vi "Initialize Waveforms V4.vi"(0 "Image Acquisition Parameters":T2={"Scan Type"=enum."Sample Scanning", "Scan Mode"=enum."XY", "Fast Axis Frequency (Hz)"=100.0, "Image Format"=128, "Line Accumulations"=1, "Frames Per Capture"=1, "Frames Accumulations"=1, "Image Dimension (um)"=[], "Number of Z Steps"=1, "Z Steps Size (um)"=1.0, "Pixel Size (nm)"=[]} {"Z Steps Size (um)" min=0.0; "Number of Z Steps" min=1; "Frames Accumulations" min=1; "Frames Per Capture" min=1; "Line Accumulations" min=1; "Image Format" items=["64 x 64"=64, "128 x 128"=128, "256 x 256"=256, "512 x 512"=512, "1024 x 1024"=1024, "2048 x 2048"=2048]}) -> (4 "Waveform Data to FPGA":T1)   [LabVIEW 2016]
uses:
  Type Defs/Image Acquisition Parameters.ctl
  Waveform Data.ctl
panel:
  in  "Slow Axis 2 Delay (Galvo - Not YZ)":i32=2
  in  "Number Data of Points":i32=5000
  # "Copyright (C) 2020 Edward S Allgeyer\n\nRedistribution and use in source and binary forms, with or without\nmodification, are permitted provided that the following conditions\nare met:\n\n1. Redistributions of source code must retain the above copyright\n   notice, this list of conditions and the following disclaimer.\n\n2. Redistributions in binary form must reproduce the above copyright\n   notice, this list of conditions and the following disclaimer in\n   the documentation and/or other materials provided with the\n   distribution.\n\n3. Neither the name of the copyright holder nor the names of its\n   contributors may be used to endorse or promote products derived\n   from this software without specific prior written permission.\n\nTHIS SOFTWARE IS PROVIDED BY THE COPYRIGHT HOLDERS AND CONTRIBUTORS\n\"AS IS\" AND ANY EXPRESS OR IMPLIED WARRANTIES, INCLUDING, BUT NOT\nLIMITED TO, THE IMPLIED WARRANTIES OF MERCHANTABILITY AND FITNESS\nFOR A PARTICULAR PURPOSE ARE DISCLAIMED. IN NO EVENT SHALL THE\nCOPYRIGHT HOLDER OR CONTRIBUTORS BE LIABLE FOR ANY DIRECT, INDIRECT,\nINCIDENTAL, SPECIAL, EXEMPLARY, OR CONSEQUENTIAL DAMAGES (INCLUDING,\nBUT NOT LIMITED TO, PROCUREMENT OF SUBSTITUTE GOODS OR SERVICES;\nLOSS OF USE, DATA, OR PROFITS; OR BUSINESS INTERRUPTION) HOWEVER\nCAUSED AND ON ANY THEORY OF LIABILITY, WHETHER IN CONTRACT, STRICT\nLIABILITY, OR TORT (INCLUDING NEGLIGENCE OR OTHERWISE) ARISING IN\nANY WAY OUT OF THE USE OF THIS SOFTWARE, EVEN IF ADVISED OF THE\nPOSSIBILITY OF SUCH DAMAGE."
  # "XY"
  # "Z"
  # "Length"
  # "Height"
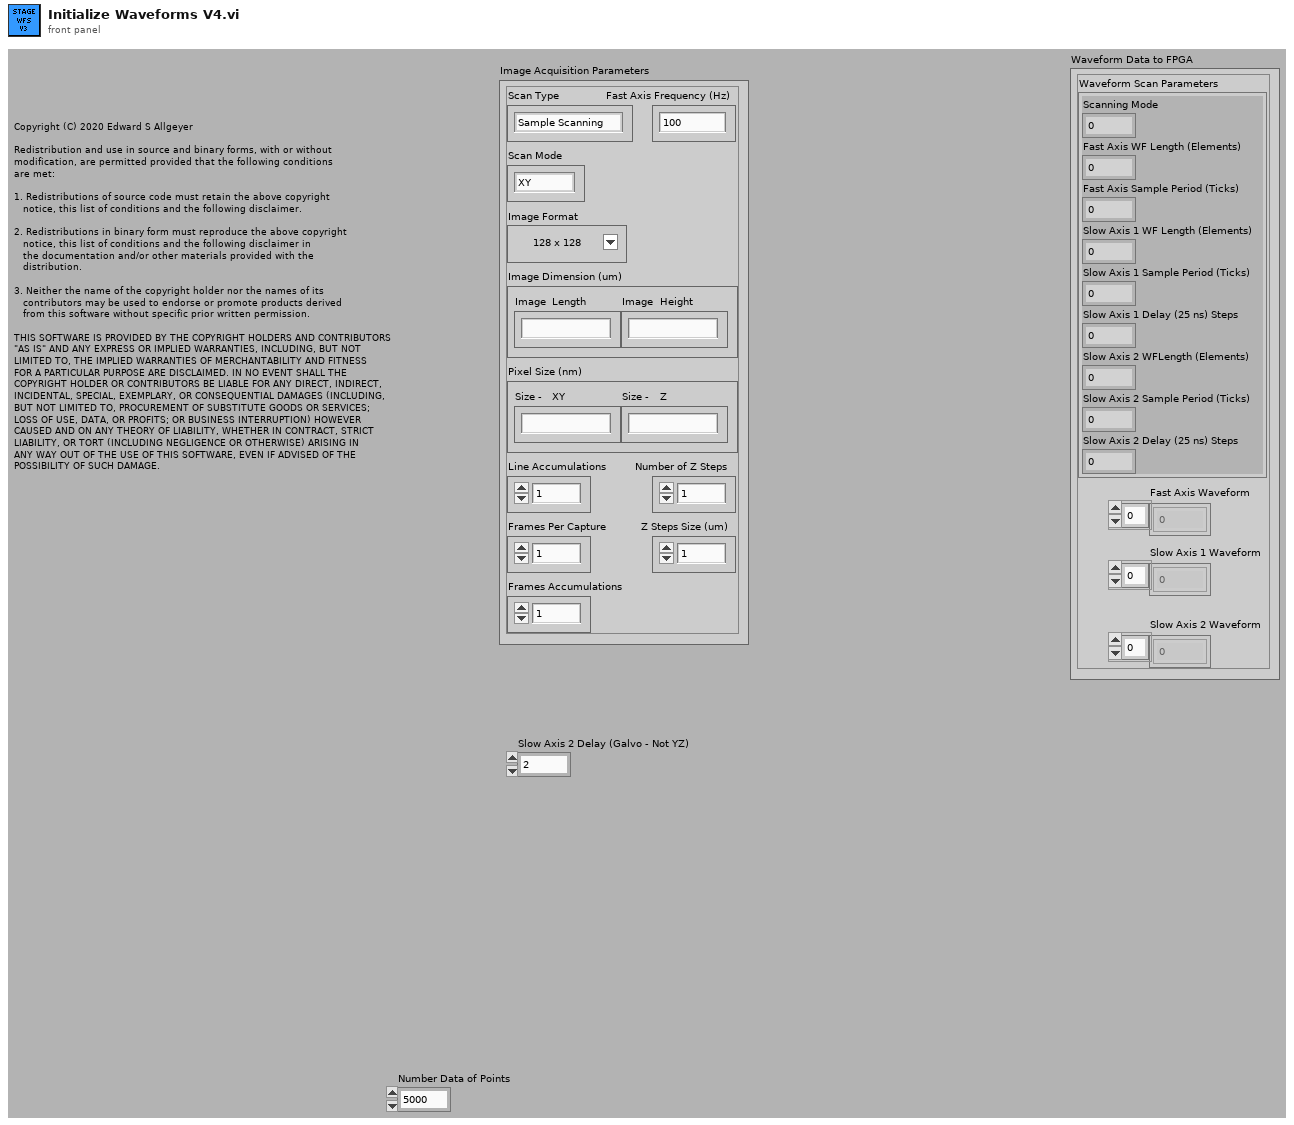
[diagram p1: front panel]
types:
  T1 = typedef "Waveform Data.ctl" = cluster{"Waveform Scan Parameters":cluster{"Scanning Mode":u8, "Fast Axis WF Length (Elements)":i32, "Fast Axis Sample Period (Ticks)":u32, "Slow Axis 1 WF Length (Elements)":i32, "Slow Axis 1 Sample Period (Ticks)":u32, "Slow Axis 1 Delay (25 ns) Steps":i32, "Slow Axis 2 WFLength (Elements)":i32, "Slow Axis 2 Sample Period (Ticks)":u32, "Slow Axis 2 Delay (25 ns) Steps":i32}, "Fast Axis Waveform":dbl[], "Slow Axis 1 Waveform":dbl[], "Slow Axis 2 Waveform":dbl[]}
  T2 = typedef "Image Acquisition Parameters.ctl" = cluster{"Scan Type":enum16{"Sample Scanning", "Beam Scanning"}, "Scan Mode":enum16{"XY", "XZ", "YZ", "XYZ"}, "Fast Axis Frequency (Hz)":dbl, "Image Format":u16, "Line Accumulations":u16, "Frames Per Capture":u16, "Frames Accumulations":u16, "Image Dimension (um)":dbl[], "Number of Z Steps":u8, "Z Steps Size (um)":dbl, "Pixel Size (nm)":dbl[]}
  T3 = cluster{"Scanning Mode":u8, "Fast Axis WF Length (Elements)":i32, "Fast Axis Sample Period (Ticks)":u32, "Slow Axis 1 WF Length (Elements)":i32, "Slow Axis 1 Sample Period (Ticks)":u32, "Slow Axis 1 Delay (25 ns) Steps":i32, "Slow Axis 2 WFLength (Elements)":i32, "Slow Axis 2 Sample Period (Ticks)":u32, "Slow Axis 2 Delay (25 ns) Steps":i32}
  T4 = typedef "Scan Parameters.ctl" = cluster{"Fast_Ax_Amp_V":dbl, "Fast_Ax_Off_V":dbl, "Slow_Ax_Amp_V":dbl, "Slow_Ax_Off_V ":dbl, "Slow_Ax_Max_V_VperS":dbl, "Slow_Ax1_Del25ns":i32, "Slow_Ax2_Del25ns":i32, "Stage_X_Off_V":dbl, "Stage_Y_Off_V":dbl, "Stage_Z_Off_V":dbl, "Galvo1_Off_V":dbl, "Galvo2_Off_V":dbl, "Last_Scan_Mode":enum16{"XY", "XZ", "YZ", "XYZ"}, "Current_Scan_Mode":enum16{"XY", "XZ", "YZ", "XYZ"}, "Fly_Back_Lines":u16, "Linear_Ramp_End":u32, "Z_Step_I16":i16, "Z_Start_I16":i16, "Laser_States _U32":u32, "590_Voltage_I16":i16, "775_AOM_Volt_I16":i16, "Blanking OFF":bool, "Unused_Axis_I16":i16}
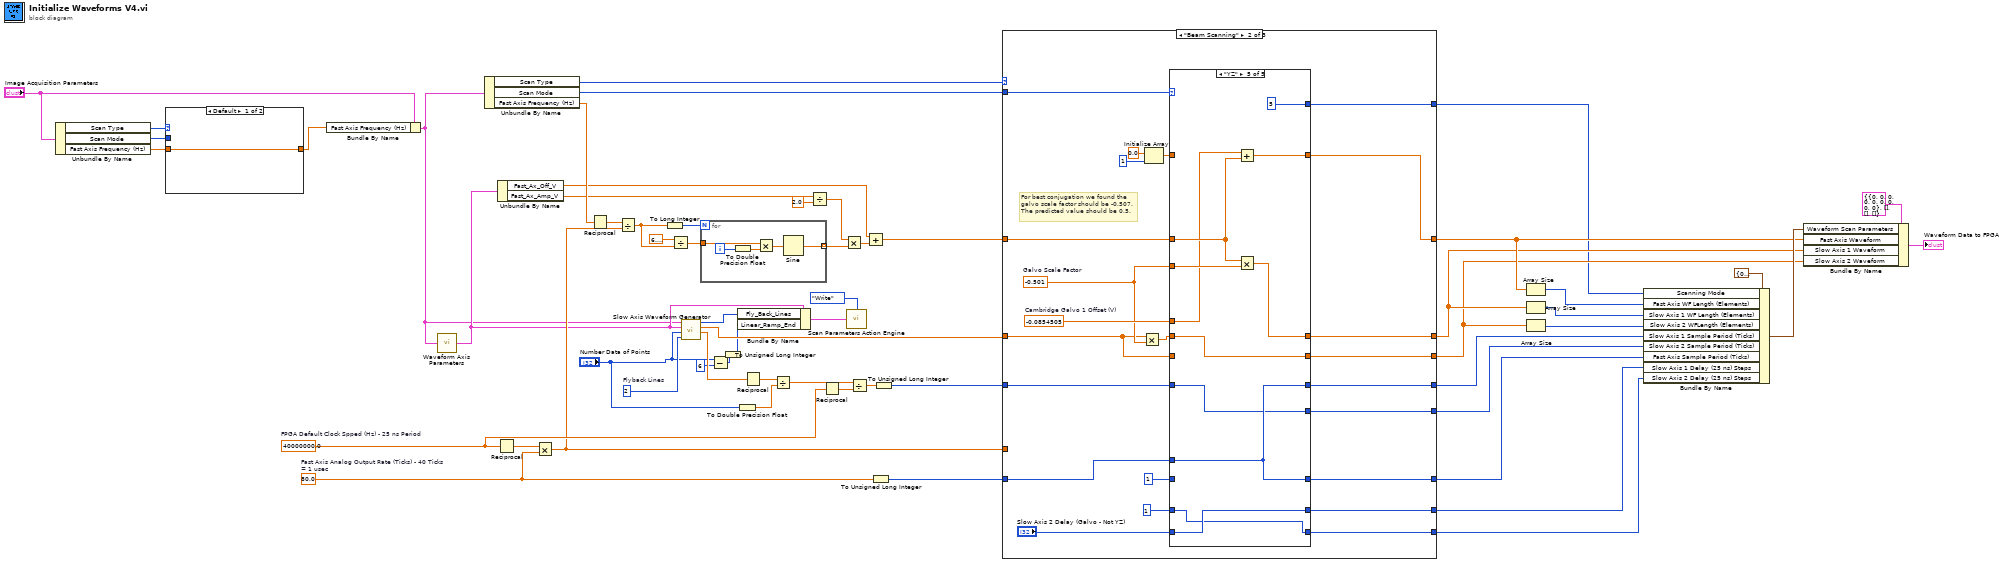
[diagram p0: block diagram]
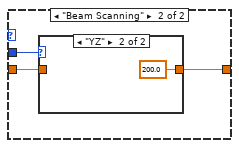
[diagram p2: hidden frame]
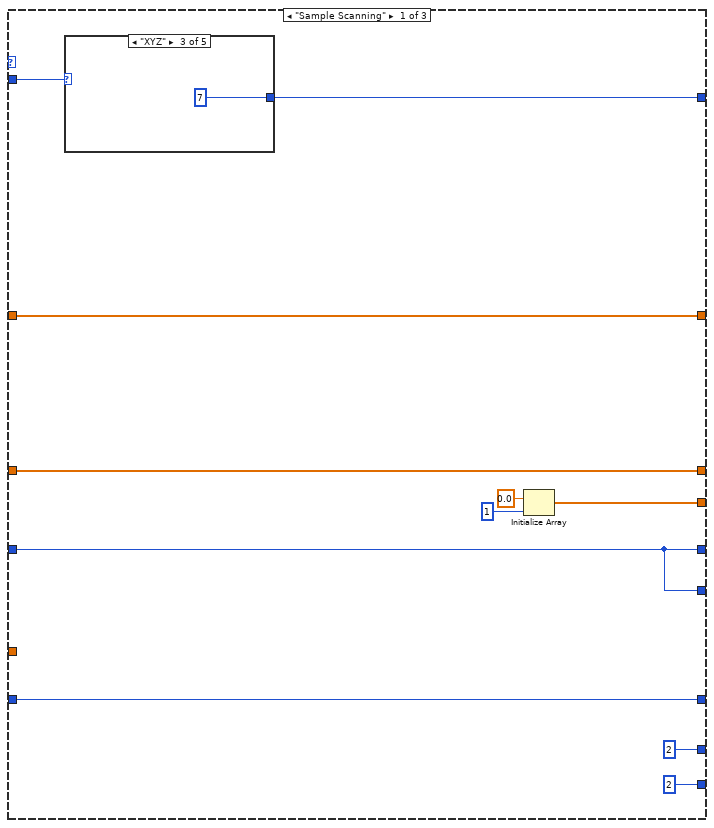
[diagram p4: hidden frame]
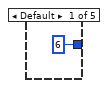
[diagram p5: hidden frame]
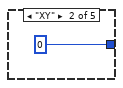
[diagram p6: hidden frame]
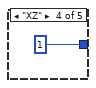
[diagram p7: hidden frame]
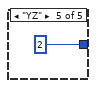
[diagram p8: hidden frame]
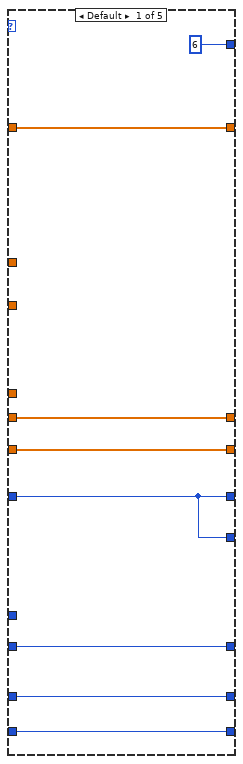
[diagram p9: hidden frame]
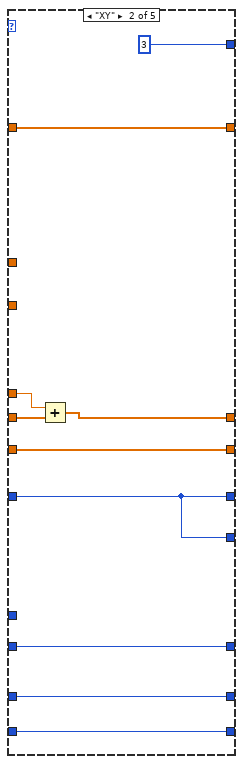
[diagram p10: hidden frame]
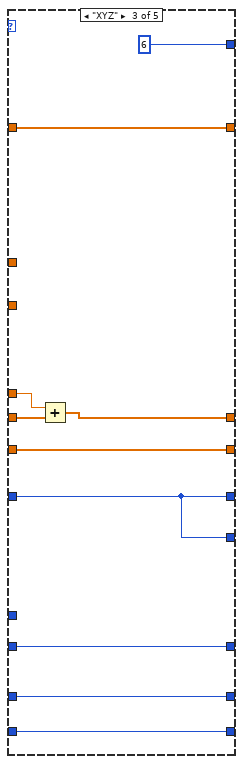
[diagram p11: hidden frame]
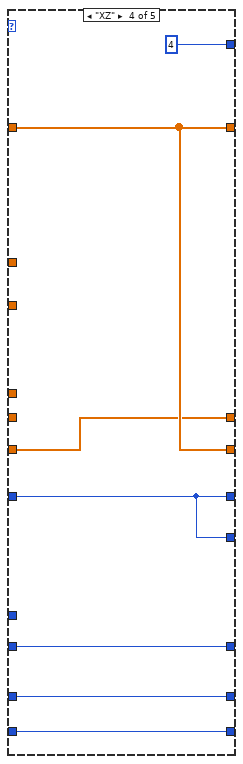
[diagram p12: hidden frame]
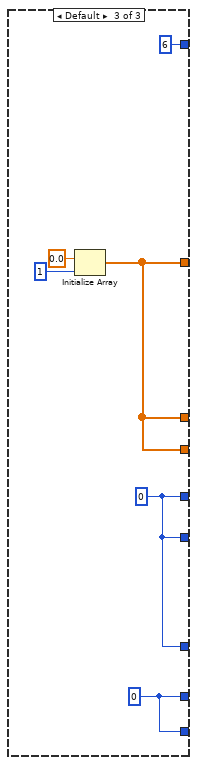
[diagram p13: hidden frame]
diagram:
  w51 = u16 2  # Flyback Lines
  w35 = 80.0  # Fast Axis Analog Output Rate (Ticks) - 40 Ticks = 1 usec
  w45 = 40000000.0  # FPGA Default Clock Spped (Hz) - 25 ns Period
  n1 = Unbundle By Name("Image Acquisition Parameters") -> ("Scan Type"=w10:enum16{"Sample Scanning", "Beam Scanning"}, "Scan Mode"=w9:enum16{"XY", "XZ", "YZ", "XYZ"}, "Fast Axis Frequency (Hz)"=w8:dbl)
  n2 = case shown="Default" w10 {
    tunnel: w9 -> [_ w63]
    tunnel: [w60 w61] -> w7
    tunnel: w8 -> [w60 w62]
    frame Default {
    }
    frame "Beam Scanning" {
      n3 = case shown="\"YZ\"" w63 {
        tunnel: [w64 200.0 ("Fast Axis Frequency (Hz)")] -> w61
        tunnel: w62 -> [w64 _]
        frame Default {
        }
        frame "YZ" {
        }
      }
    }
  }
  n4 = Bundle By Name(cluster="Image Acquisition Parameters", "Fast Axis Frequency (Hz)"=w7) -> (w5:T2)
  n5 = call "Waveform Axis Parameters.vi"("Image Acquisition Parameters"=w5) -> ("Scan Parameters"=w11:T4)  [unwired: 14 in]
  n6 = Unbundle By Name(w5) -> ("Scan Type"=w50:enum16{"Sample Scanning", "Beam Scanning"}, "Scan Mode"=w49:enum16{"XY", "XZ", "YZ", "XYZ"}, "Fast Axis Frequency (Hz)"=w20:dbl)
  n7 = Unbundle By Name(w11) -> ("Fast_Ax_Off_V"=w17:dbl, "Fast_Ax_Amp_V"=w18:dbl)
  n8 = Reciprocal(x=w45) -> (1/x=w48:dbl)
  n9 = Multiply(x=w48, y=w35) -> (x*y=w15:dbl)
  n10 = Reciprocal(x=w20) -> (1/x=w25:dbl)
  n11 = Divide(x=w25, y=w15) -> (x/y=w23:dbl)
  n12 = To Long Integer(number=w23) -> (32bit integer=w24:i32)
  n13 = Divide(x=6.283185307179586, y=w23) -> (x/y=w28:dbl)
  n14 = call "Slow Axis Waveform Generator.vi"("Flyback Lines"=w51, "Number Data of Points"="Number Data of Points", "Scan Parameters"=w11, "Image Acquisition Parameters"=w5) -> ("Slow Axis Frequency"=w46:dbl, "Slow Axis Waveform"=w47:dbl[], "Flyback Lines"=w14:u16)  [unwired: 1 out]
  n15 = for {
    N: w24 -> [_]
    tunnel: w28 -> [w70]
    tunnel: [w67] -> w27 mode=indexing
    i -> [w66]
    n16 = To Double Precision Float(number=w66) -> (double precision float=w69:dbl)
    n17 = Multiply(x=w70, y=w69) -> (x*y=w68:dbl)
    n18 = Sine(x=w68) -> (sin(x)=w67:dbl)
  }
  n19 = Subtract(x="Number Data of Points", y=6) -> (x-y=w2:i32)
  n20 = To Unsigned Long Integer(number=w2) -> (unsigned 32bit integer=w1:u32)
  n21 = Bundle By Name(cluster=w11, "Fly_Back_Lines"=w14, "Linear_Ramp_End"=w1) -> (w12:T4)
  n22 = To Double Precision Float(number="Number Data of Points") -> (double precision float=w55:dbl)
  n23 = Reciprocal(x=w46) -> (1/x=w56:dbl)
  n24 = Divide(x=w56, y=w55) -> (x/y=w54:dbl)
  n25 = Divide(x=w18, y=2.0) -> (x/y=w21:dbl)
  n26 = Reciprocal(x=w45) -> (1/x=w53:dbl)
  n27 = Multiply(x=w21, y=w27) -> (x*y=w26:dbl[])
  n28 = call "Scan Parameters Action Engine.vi"("Action"=enum16{"Read", "Write"}."Write", "Scan Parameters IN"=w12) -> ()  [unwired: 13 in, 1 out]
  n29 = Divide(x=w54, y=w53) -> (x/y=w52:dbl)
  n30 = Add(x=w17, y=w26) -> (x+y=w19:dbl[])
  n31 = To Unsigned Long Integer(number=w35) -> (unsigned 32bit integer=w34:u32)
  n32 = To Unsigned Long Integer(number=w52) -> (unsigned 32bit integer=w44:u32)
  n33 = case shown="\"Beam Scanning\"" w50 {
    tunnel: w49 -> [w81 w109 _]
    tunnel: w15 -> [_ _ _]
    tunnel: [w71 w107 w158] -> w42
    tunnel: w47 -> [w80 w87 _]
    tunnel: [w80 w103 w158] -> w41
    tunnel: [w77 w102 w158] -> w40
    tunnel: w44 -> [w74 w93 _]
    tunnel: [w76 w108 u8 6 ("Scanning Mode")] -> w36
    tunnel: w34 -> [w75 w90 _]
    tunnel: [w75 w99 w157] -> w33
    tunnel: [w74 w92 w157] -> w32
    tunnel: [w74 w91 w157] -> w31
    tunnel: [2 ("Slow Axis 2 Delay (25 ns) Steps") w98 w156] -> w30
    tunnel: [2 ("Slow Axis 2 Delay (25 ns) Steps") w96 w156] -> w16
    tunnel: w19 -> [w71 w100 _]
    frame "Sample Scanning" {
      n34 = case shown="\"XYZ\"" w81 {
        tunnel: [u8 6 ("Scanning Mode") u8 0 ("Scanning Mode") u8 7 ("Scanning Mode") u8 1 ("Scanning Mode") u8 2 ("Scanning Mode")] -> w76
        frame Default {
        }
        frame "XY" {
        }
        frame "XYZ" {
        }
        frame "XZ" {
        }
        frame "YZ" {
        }
      }
      n35 = Initialize Array(0.0 ("element"), 1 ("dimension size")) -> (w77:dbl[])
    }
    frame "Beam Scanning" {
      w88 = -0.501  # Galvo Scale Factor
      w101 = -0.0854505  # Cambridge Galvo 1 Offset (V)
      # "For best conjugation we found the\ngalvo scale factor should be -0.507.\nThe predicted value should be 0.5."
      n36 = Multiply(x=w87, y=w88) -> (x*y=w89:dbl[])
      n37 = Initialize Array(0.0 ("element"), 1 ("dimension size")) -> (w104:dbl[])
      n38 = case shown="\"YZ\"" w109 {
        tunnel: [u8 6 ("Scanning Mode") u8 3 ("Scanning Mode") u8 6 ("Scanning Mode") u8 4 ("Scanning Mode") u8 5 ("Scanning Mode")] -> w108
        tunnel: [w116 w126 w136 w143 w149] -> w107
        tunnel: w104 -> [w116 w126 w136 w143 _]
        tunnel: [w115 w123 w133 w138 w153] -> w103
        tunnel: w89 -> [w115 w124 w134 _ w154]
        tunnel: w87 -> [w114 w125 w135 w138 _]
        tunnel: [w114 w125 w135 w143 w154] -> w102
        tunnel: w101 -> [_ w122 w132 _ w150]
        tunnel: w100 -> [_ _ _ _ w151]
        tunnel: w88 -> [_ _ _ _ w152]
        tunnel: [w113 w121 w131 w141 w147] -> w99
        tunnel: u32 1 -> [w113 w121 w131 w141 _]
        tunnel: [w111 w120 w130 w139 w145] -> w98
        tunnel: "Slow Axis 2 Delay (Galvo - Not YZ)" -> [w111 w120 w130 w139 w148]
        tunnel: [w112 w119 w129 w140 w148] -> w96
        tunnel: 1 ("Slow Axis 1 Delay (25 ns) Steps") -> [w112 w119 w129 w140 w145]
        tunnel: [w110 w118 w128 w142 w147] -> w92
        tunnel: w93 -> [w110 w118 w128 w142 w146]
        tunnel: [w110 w118 w128 w142 w146] -> w91
        tunnel: w90 -> [_ _ _ _ w147]
        frame Default {
        }
        frame "XY" {
          n39 = Add(x=w122, y=w124) -> (x+y=w123:dbl[])
        }
        frame "XYZ" {
          n40 = Add(x=w132, y=w134) -> (x+y=w133:dbl[])
        }
        frame "XZ" {
        }
        frame "YZ" {
          n41 = Add(x=w150, y=w151) -> (x+y=w149:dbl[])
          n42 = Multiply(x=w151, y=w152) -> (x*y=w153:dbl[])
        }
      }
    }
    frame Default {
      w156 = 0 ("Slow Axis 2 Delay (25 ns) Steps")
      w157 = u32 0
      n43 = Initialize Array(0.0 ("element"), 1 ("dimension size")) -> (w158:dbl[])
    }
  }
  n44 = Array Size(array=w42) -> (size(s)=w39:i32)
  n45 = Array Size(array=w41) -> (size(s)=w38:i32)
  n46 = Array Size(array=w40) -> (size(s)=w37:i32)
  n47 = Bundle By Name(cluster=T3 {"Scanning Mode"=0, "Fast Axis WF Length (Elements)"=0, "Fast Axis Sample Period (Ticks)"=0, "Slow Axis 1 WF Length (Elements)"=0, "Slow Axis 1 Sample Period (Ticks)"=0, "Slow Axis 1 Delay (25 ns) Steps"=0, "Slow Axis 2 WFLength (Elements)"=0, "Slow Axis 2 Sample Period (Ticks)"=0, "Slow Axis 2 Delay (25 ns) Steps"=0} ("Waveform Scan Parameters"), "Scanning Mode"=w36, "Fast Axis WF Length (Elements)"=w39, "Slow Axis 1 WF Length (Elements)"=w38, "Slow Axis 2 WFLength (Elements)"=w37, "Slow Axis 1 Sample Period (Ticks)"=w32, "Slow Axis 2 Sample Period (Ticks)"=w31, "Fast Axis Sample Period (Ticks)"=w33, "Slow Axis 1 Delay (25 ns) Steps"=w16, "Slow Axis 2 Delay (25 ns) Steps"=w30) -> (w43:T3)
  n48 = Bundle By Name(cluster=T1 {"Waveform Scan Parameters"={"Scanning Mode"=0, "Fast Axis WF Length (Elements)"=0, "Fast Axis Sample Period (Ticks)"=0, "Slow Axis 1 WF Length (Elements)"=0, "Slow Axis 1 Sample Period (Ticks)"=0, "Slow Axis 1 Delay (25 ns) Steps"=0, "Slow Axis 2 WFLength (Elements)"=0, "Slow Axis 2 Sample Period (Ticks)"=0, "Slow Axis 2 Delay (25 ns) Steps"=0}, "Fast Axis Waveform"=[], "Slow Axis 1 Waveform"=[], "Slow Axis 2 Waveform"=[]} ("Waveform Data"), "Waveform Scan Parameters"=w43, "Fast Axis Waveform"=w42, "Slow Axis 1 Waveform"=w41, "Slow Axis 2 Waveform"=w40) -> (→"Waveform Data to FPGA":T1)
